vi "Expand Bounds 2D.vi"(10 "Tolerance (N)":dbl, 11 "Entry":T1[](array[typedef]) {"Axial Force" format="%.4f"; "Lateral Force" format="%.4f"}) -> (0 "Bottom Left":T1 {"Axial Force" format="%.4f"; "Lateral Force" format="%.4f"}, 1 "Bottom Right":T1 {"Axial Force" format="%.4f"; "Lateral Force" format="%.4f"}, 2 "Top Right":T1 {"Axial Force" format="%.4f"; "Lateral Force" format="%.4f"}, 3 "Top Left":T1 {"Axial Force" format="%.4f"; "Lateral Force" format="%.4f"})   [LabVIEW 2016, in "Test Actuator State.lvclass"]
uses:
  Test Actuator State.lvclass
  Typedefs/ForcePair.ctl
  Typedefs/FAMT Typedefs.lvlib
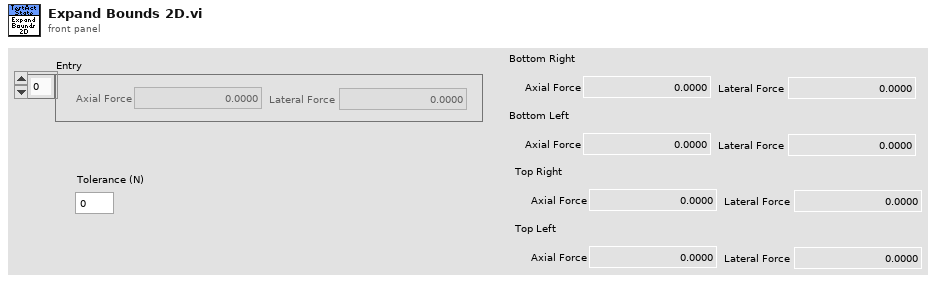
[diagram p1: front panel]
types:
  T1 = typedef "FAMT Typedefs.lvlib/ForcePair.ctl" = cluster{"Axial Force":dbl, "Lateral Force":dbl}
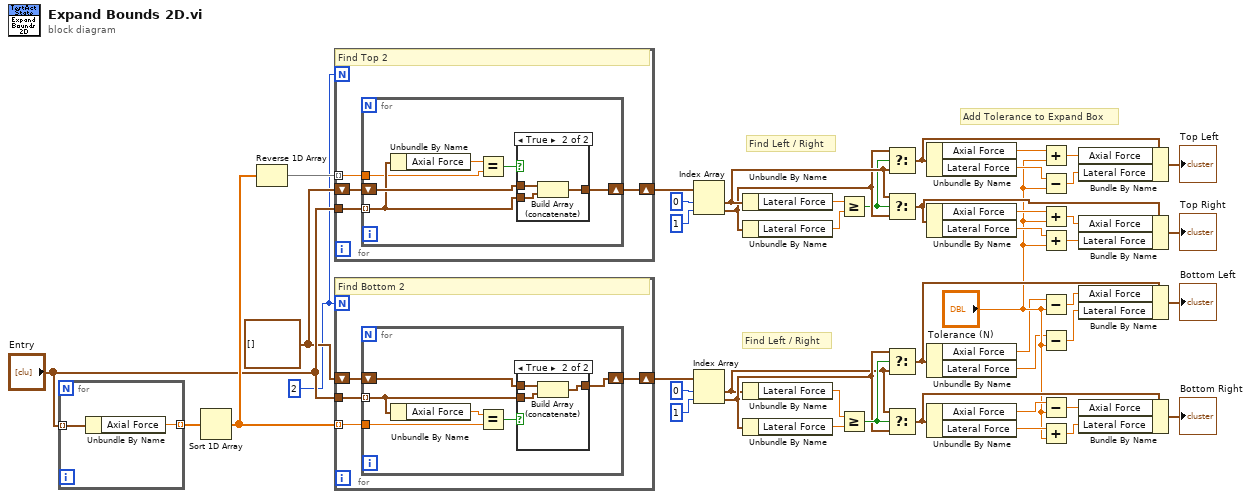
[diagram p0: block diagram]
diagram:
  w43 = T1[] []
  w1 = 2
  # "Add Tolerance to Expand Box"
  # "Find Left / Right"
  # "Find Left / Right"
  n1 = for {
    tunnel: "Entry" -> [w49] mode=indexing
    tunnel: [w48] -> w47 mode=indexing
    n2 = Unbundle By Name(w49) -> ("Axial Force"=w48:dbl)
  }
  n3 = Sort 1D Array(array=w47) -> (sorted array=w45:dbl[])
  n4 = Reverse 1D Array(array=w45) -> (reversed array=w46:dbl[])
  n5 = for {
    N: w1 -> [_]
    tunnel: "Entry" -> [w53]
    tunnel: w46 -> [w50] mode=indexing
    shift-right: [w52] -> w27
    shift-left: w43 -> [w51]
    # "Find Top 2"
    n6 = for {
      tunnel: w53 -> [w57] mode=indexing
      shift-right: [w59] -> w52
      shift-left: w51 -> [w58]
      tunnel: w50 -> [w55]
      n7 = Unbundle By Name(w57) -> ("Axial Force"=w56:dbl)
      n8 = Equal?(x=w56, y=w55) -> (x = y?=w54:bool)
      n9 = case shown="True" w54 {
        tunnel: w57 -> [_ w63]
        tunnel: [w60 w62] -> w59
        tunnel: w58 -> [w60 w61]
        frame False {
        }
        frame True {
          n10 = Build Array (concatenate)(w61, w63) -> (w62:T1[])
        }
      }
    }
  }
  n11 = for {
    N: w1 -> [_]
    tunnel: "Entry" -> [w67]
    tunnel: w45 -> [w64] mode=indexing
    shift-right: [w66] -> w40
    shift-left: w43 -> [w65]
    # "Find Bottom 2"
    n12 = for {
      tunnel: w67 -> [w71] mode=indexing
      shift-right: [w73] -> w66
      shift-left: w65 -> [w72]
      tunnel: w64 -> [w69]
      n13 = Unbundle By Name(w71) -> ("Axial Force"=w70:dbl)
      n14 = Equal?(x=w70, y=w69) -> (x = y?=w68:bool)
      n15 = case shown="True" w68 {
        tunnel: w71 -> [_ w77]
        tunnel: [w74 w76] -> w73
        tunnel: w72 -> [w74 w75]
        frame False {
        }
        frame True {
          n16 = Build Array (concatenate)(w75, w77) -> (w76:T1[])
        }
      }
    }
  }
  n17 = Index Array(array=w27, index #1=0 ("index"), index #2=1 ("index")) -> (element #1=w34:T1, element #2=w33:T1)
  n18 = Index Array(array=w40, index #1=0 ("index"), index #2=1 ("index")) -> (element #1=w35:T1, element #2=w36:T1)
  n19 = Unbundle By Name(w34) -> ("Lateral Force"=w30:dbl)
  n20 = Unbundle By Name(w33) -> ("Lateral Force"=w31:dbl)
  n21 = Unbundle By Name(w35) -> ("Lateral Force"=w39:dbl)
  n22 = Unbundle By Name(w36) -> ("Lateral Force"=w38:dbl)
  n23 = Greater Or Equal?(x=w30, y=w31) -> (x >= y?=w32:bool)
  n24 = Greater Or Equal?(x=w39, y=w38) -> (x >= y?=w37:bool)
  n25 = Select(t=w33, s=w32, f=w34) -> (s? t:f=w21:T1)
  n26 = Select(t=w34, s=w32, f=w33) -> (s? t:f=w26:T1)
  n27 = Select(t=w36, s=w37, f=w35) -> (s? t:f=w9:T1)
  n28 = Select(t=w35, s=w37, f=w36) -> (s? t:f=w14:T1)
  n29 = Unbundle By Name(w21) -> ("Axial Force"=w17:dbl, "Lateral Force"=w19:dbl)
  n30 = Unbundle By Name(w26) -> ("Axial Force"=w23:dbl, "Lateral Force"=w24:dbl)
  n31 = Unbundle By Name(w9) -> ("Axial Force"=w3:dbl, "Lateral Force"=w2:dbl)
  n32 = Unbundle By Name(w14) -> ("Axial Force"=w13:dbl, "Lateral Force"=w12:dbl)
  n33 = Add(x=w17, y="Tolerance (N)") -> (x+y=w16:dbl)
  n34 = Subtract(x=w19, y="Tolerance (N)") -> (x-y=w18:dbl)
  n35 = Add(x=w23, y="Tolerance (N)") -> (x+y=w22:dbl)
  n36 = Add(x=w24, y="Tolerance (N)") -> (x+y=w7:dbl)
  n37 = Subtract(x=w3, y="Tolerance (N)") -> (x-y=w5:dbl)
  n38 = Subtract(x=w2, y="Tolerance (N)") -> (x-y=w6:dbl)
  n39 = Subtract(x=w13, y="Tolerance (N)") -> (x-y=w10:dbl)
  n40 = Add(x=w12, y="Tolerance (N)") -> (x+y=w11:dbl)
  n41 = Bundle By Name(cluster=w21, "Axial Force"=w16, "Lateral Force"=w18) -> (→"Top Left":T1)
  n42 = Bundle By Name(cluster=w26, "Axial Force"=w22, "Lateral Force"=w7) -> (→"Top Right":T1)
  n43 = Bundle By Name(cluster=w9, "Axial Force"=w5, "Lateral Force"=w6) -> (→"Bottom Left":T1)
  n44 = Bundle By Name(cluster=w14, "Axial Force"=w10, "Lateral Force"=w11) -> (→"Bottom Right":T1)
